vi "Init.vi"(7 "Prevent Cache (T)":bool=TRUE, 8 "error in (no error)":errorcluster, 10 "Godot Export HTML":path, 11 "Port (10027)":u16=10027) -> (0 "error out":errorcluster, 3 "GodotServer out":refnum<class "GodotServer.lvclass">)   [LabVIEW 2020, in "GodotLV.lvlib" / "GodotServer.lvclass"]
doc: "Initializes the web server for the specified page to be loaded and it will be listening on the specified port. The server will not be active until <b>Start Server.vi</b> is called.\n\nEnsure to call <b>Cleanup.vi</b> when done to release all resources for the server."
uses:
  GodotServer.lvclass
  GodotServer.lvclass/GodotServer.ctl
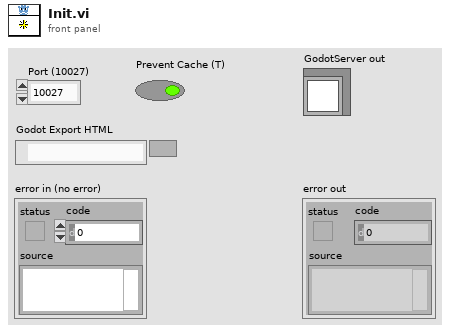
[diagram p1: front panel]
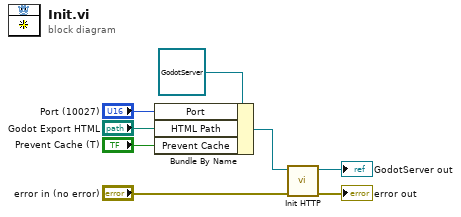
[diagram p0: block diagram]
diagram:
  n1 = Bundle By Name(cluster=refnum<class "GodotServer.lvclass"> refnum ("GodotServer in"), "Port"="Port (10027)", "HTML Path"="Godot Export HTML", "Prevent Cache"="Prevent Cache (T)") -> (w3:refnum<class "GodotServer.lvclass">)
  n2 = call "Init HTTP.vi"("error in (no error)"="error in (no error)", "GodotServer in"=w3) -> ("error out"=→"error out":errorcluster, "GodotServer out"=→"GodotServer out":refnum<class "GodotServer.lvclass">)  [unwired: 8 in]
